vi "Write X-offsets.vi"(8 "error in (no error)":errorcluster, 10 "X-offsets":i32[](array[numeric]), 11 "Configuration in":refnum<class "CV-Configuration.lvclass">) -> (0 "error out":errorcluster, 3 "Configuration out":refnum<class "CV-Configuration.lvclass">)   [LabVIEW 2013, in "CameraVision.lvlib" / "CV-Configuration.lvclass"]
uses:
  CV-Configuration.lvclass
  CV-Configuration.lvclass/CV-Configuration.ctl
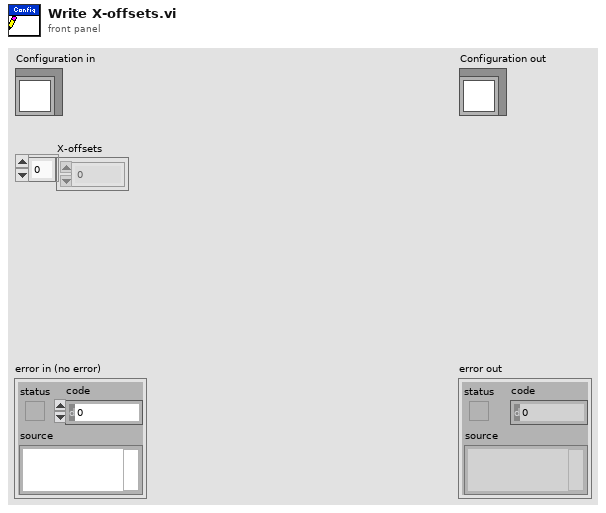
[diagram p1: front panel]
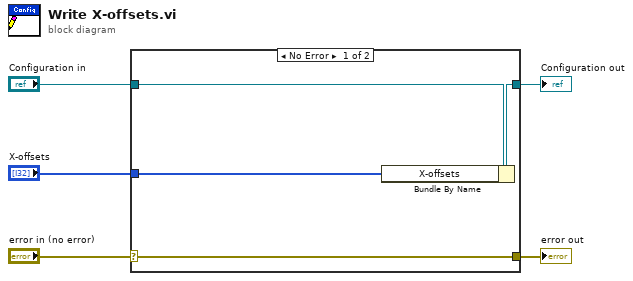
[diagram p0: block diagram]
diagram:
  n1 = case shown="No Error" "error in (no error)" {
    selector: "error in (no error)" -> [w9 w10]
    tunnel: [w9 w10] -> w4
    tunnel: [w7 w11] -> w2
    tunnel: "Configuration in" -> [w8 w11]
    tunnel: "X-offsets" -> [w6 _]
    frame No Error {
      n2 = Bundle By Name(cluster=w8, "X-offsets"=w6) -> (w7:refnum<class "CV-Configuration.lvclass">)
    }
    frame Error {
    }
  }
  "error out" <- w4
  "Configuration out" <- w2
